vi "468_lab8_ecg_sim.vi"(3 "i":i32, 4 "duration":dbl=3.0, 5 "file path":path) -> (0 "fs":dbl=360.0, 2 "signal":dbl[](graph))   [LabVIEW 2019]
uses:
  <vilib>/Utility/file.llb/Read Delimited Spreadsheet (DBL).vi
panel:
  out "size(s)":i32
  out "index":i32
  out "length":dbl
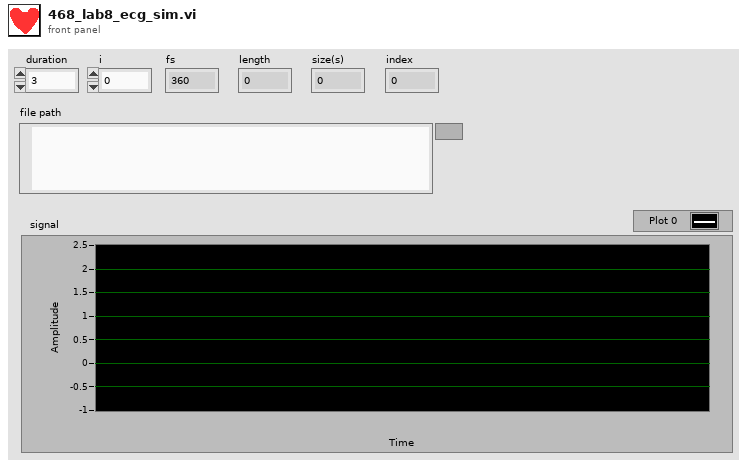
[diagram p1: front panel]
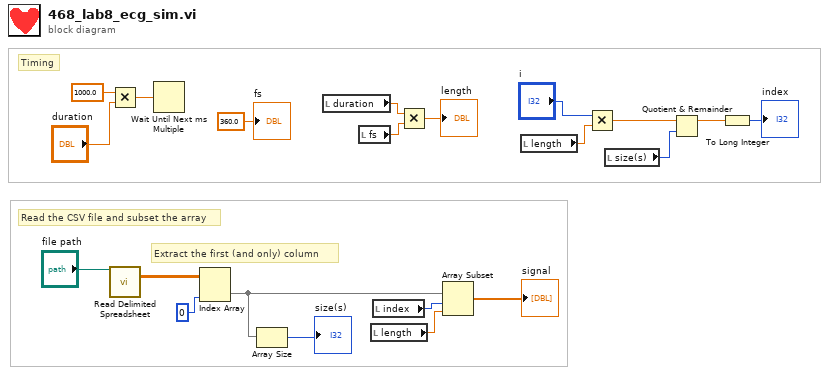
[diagram p0: block diagram]
diagram:
  # "Read the CSV file and subset the array"
  # "Timing"
  # "Extract the first (and only) column"
  n1 = Multiply(x=1000.0, y="duration") -> (x*y=w14:dbl)
  n2 = call-poly <vilib>:"Read Delimited Spreadsheet.vi"("file path (dialog if empty)"="file path") -> ("all rows"=w20:dbl[][])  [unwired: 9 in, 5 out]
  n3 = Wait Until Next ms Multiple(millisecond multiple=w14) -> ()  [unwired: 1 out]
  n4 = Index Array(array=w20, index (col)=0 ("disabled index (col)")) -> (element=w10:dbl[])  [unwired: 1 in]
  n5 = Array Size(array=w10) -> (size(s)=→"size(s)":i32)
  n6 = local read "duration"() -> (w13:dbl)
  n7 = local read "fs"() -> (w12:dbl)
  n8 = local read "length"() -> (w5:dbl)
  n9 = local read "index"() -> (w4:i32)
  n10 = Multiply(x=w13, y=w12) -> (x*y=→"length":dbl)
  n11 = Array Subset "Array Subset"(array=w10, index=w4, length=w5) -> (→"signal":dbl[])
  n12 = local read "length"() -> (w8:dbl)
  n13 = Multiply(x="i", y=w8) -> (x*y=w3:dbl)
  n14 = local read "size(s)"() -> (w2:i32)
  n15 = Quotient & Remainder(x=w3, y=w2) -> (x-y*floor(x/y)=w1:dbl)  [unwired: 1 out]
  n16 = To Long Integer(number=w1) -> (32bit integer=→"index":i32)
  "fs" <- 360.0
